vi "Read Measurement.vi"(8 "error in (no error)":errorcluster, 9 "Channel (1: Channel 1)":i32(ring)=1 items=["Channel 1"=1, "Channel 2"=2, "Channel 3"=3, "Channel 4"=4], 10 "Measurement Type (0: Frequency)":i32(ring) items=["Frequency", "Mean", "Period", "Pulse Duty", "Peak to Peak", "Cycle RMS", "Minimum", "Maximum", "Rise Time", "Fall Time", "Positive Width", "Negative Width", "Amplitude", "Cycle Mean", "High", "Low", "Negative Duty", "Positive Overshoot", "Negative Overshoot", "Cursor Mean", "Burst Width", "Positive Pulse Count", "Negative Pulse Count", "Rising Edge Count", "Falling Edge Count", "Area", "Cycle Area", "RMS", "Cursor RMS"], 11 "Osciloscope in":refnum<class "Osciloscope.lvclass">) -> (0 "error out":errorcluster, 1 "Measurement":dbl, 2 "Units":string, 3 "Osciloscope out":refnum<class "Osciloscope.lvclass">)   [LabVIEW 2020, in "Controlador.lvlib" / "Osciloscope.lvclass"]
uses:
  Osciloscope.lvclass
  Osciloscope.lvclass/Osciloscope.ctl
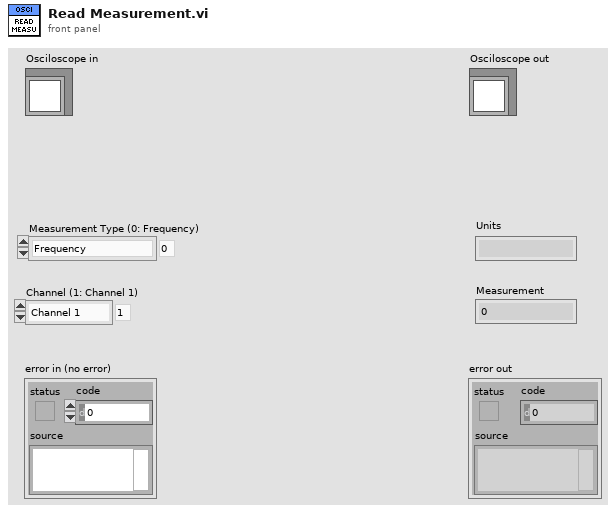
[diagram p1: front panel]
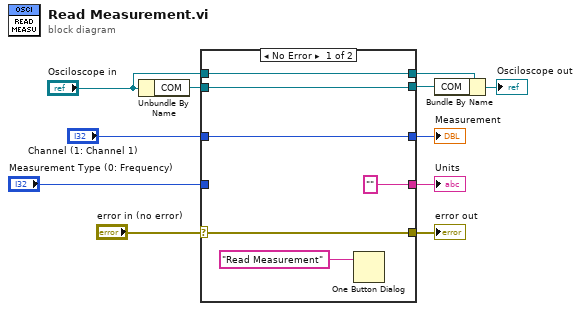
[diagram p0: block diagram]
diagram:
  n1 = Unbundle By Name("Osciloscope in") -> ("COM"=w5:refnum<visa-resource-name>)
  n2 = case shown="No Error" "error in (no error)" {
    selector: "error in (no error)" -> [w16 w19]
    tunnel: [w16 w19] -> w10
    tunnel: [w17 w18] -> w4
    tunnel: "Osciloscope in" -> [w17 w18]
    tunnel: [w15 _] -> w2
    tunnel: [w14 _] -> w9
    tunnel: w5 -> [w15 _]
    tunnel: "Channel (1: Channel 1)" -> [w14 _]
    tunnel: "Measurement Type (0: Frequency)" -> [_ _]
    tunnel: ["" ("Units") _] -> w1
    frame No Error {
      n3 = One Button Dialog(message="Read Measurement") -> ()  [unwired: 1 in, 1 out]
    }
    frame Error {
    }
  }
  "error out" <- w10
  "Units" <- w1
  "Measurement" <- w9
  n4 = Bundle By Name(cluster=w4, "COM"=w2) -> (→"Osciloscope out":refnum<class "Osciloscope.lvclass">)
